vi "Error Process.vi"(8 "error in (no error)":errorcluster, 11 "View Model":T1) -> (0 "error out":errorcluster)   [LabVIEW 2013]
doc: "Responsible for collecting and handling all errors."
uses:
  View Model/Controls/View Model.ctl
  Controls/Error Model.ctl
  Controls/Error Types.ctl
  View Model/Controls/Shared Model.ctl
  Elevator Controller/Controls/Elevator Model.ctl
  Elevator Controller/Controls/Controller Overhead.ctl
  Elevator Controller/Controls/Elevator States.ctl
  Elevator Controller/Controls/Elevator Location.ctl
  Elevator Controller/Controls/Elevator Command Event.ctl
  Elevator Controller/Controls/Elevator Commands.ctl
  Configuration/Controls/Configuration Model.ctl
  Configuration/Controls/Configuration Data.ctl
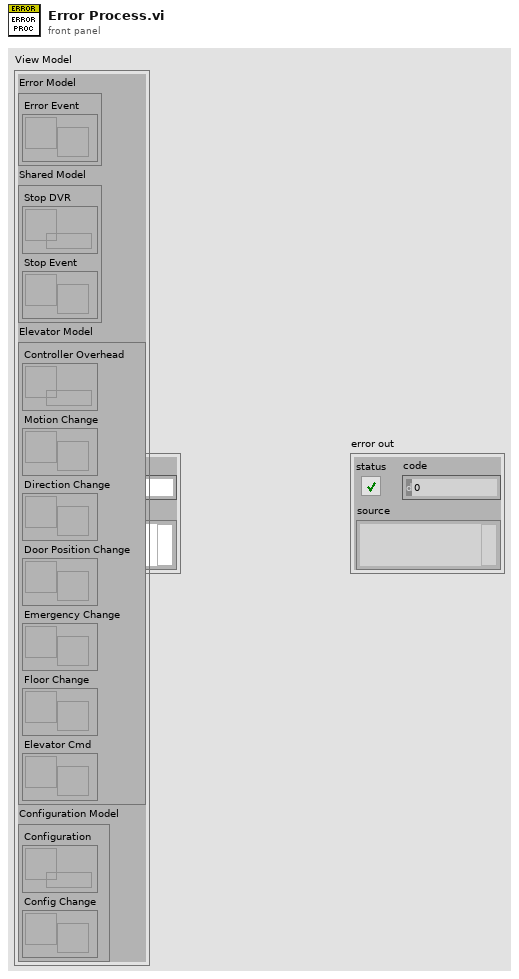
[diagram p1: front panel]
types:
  T1 = typedef "View Model.ctl" = cluster{"Error Model":T2, "Shared Model":T3, "Elevator Model":T4, "Configuration Model":T5}
  T2 = typedef "Error Model.ctl" = cluster{"Error Event":refnum<user-event>}
  T3 = typedef "Shared Model.ctl" = cluster{"Stop DVR":refnum<data-value>, "Stop Event":refnum<user-event>}
  T4 = typedef "Elevator Model.ctl" = cluster{"Controller Overhead":refnum<data-value>, "Motion Change":refnum<user-event>, "Direction Change":refnum<user-event>, "Door Position Change":refnum<user-event>, "Emergency Change":refnum<user-event>, "Floor Change":refnum<user-event>, "Elevator Cmd":refnum<user-event>}
  T5 = typedef "Configuration Model.ctl" = cluster{"Configuration":refnum<data-value>, "Config Change":refnum<user-event>}
  T6 = typedef "Error Types.ctl" = enum16{"Console Error", "Process Step Error", "Sensor Interface IO Error"}
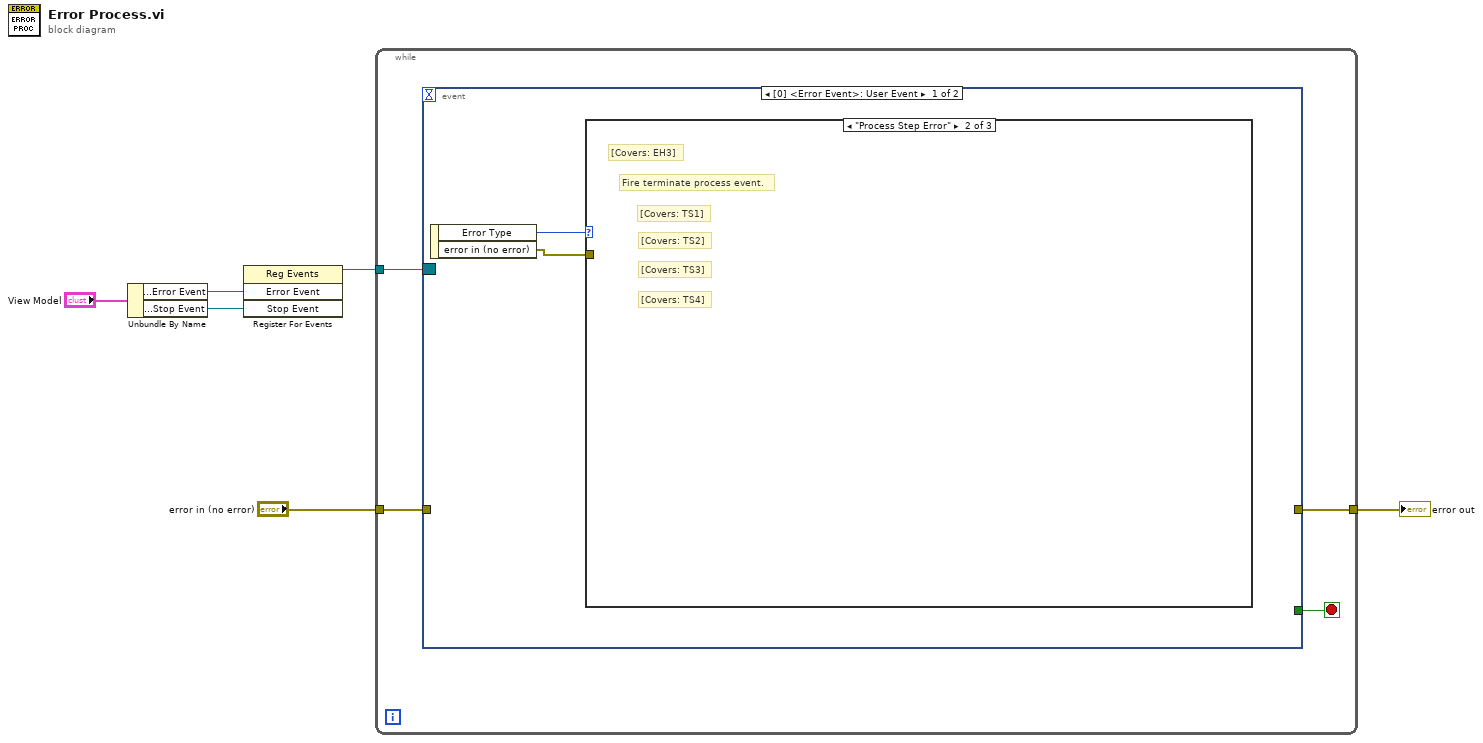
[diagram p0: block diagram]
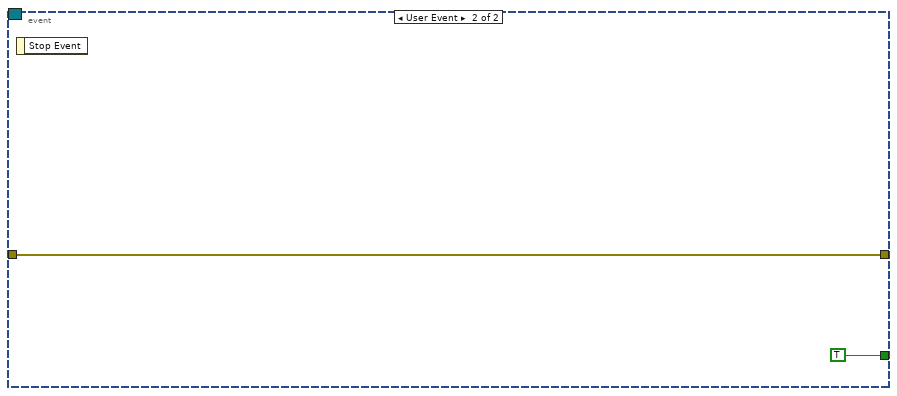
[diagram p4: hidden frame]
diagram:
  n1 = Unbundle By Name("View Model") -> ("Error Model.Error Event"=w5:refnum<user-event>, "Shared Model.Stop Event"=w3:refnum<user-event>)
  n2 = register-events(w5, w3) -> (reference out=w4:refnum<event-registration>)  [unwired: 2 in, 1 out]
  n3 = while {
    tunnel: w4 -> [w10]
    tunnel: "error in (no error)" -> [w8]
    tunnel: [w7] -> w1
    stop <- w9 stop-if-true
    n4 = event shown="[0] <Error Event>: User Event" {
      selector: w10 -> [_ _]
      dyn-events: _ -> [_ _]
      timeout: _ -> [_ _]
      tunnel: [_ TRUE] -> w9
      tunnel: w8 -> [_ w13]
      tunnel: [_ w13] -> w7
      event User Event {
        n5 = event-data() -> ("Error Type"=w12:T6, "error in (no error)"=w11:errorcluster)  [unwired: 1 in]
        n6 = case shown="\"Process Step Error\"" w12 {
          tunnel: w11 -> [_ _ _]
          frame "Console Error", Default {
            # "[Covers: EH1]"
            # "[Covers: EH1B]"
            # "[Covers: EH1A]"
            # "Console Error: Alert user.\nIf error source = Display Console View, notify user and clear\nerror.\n\nIf error source = User Console View, Allow user to choose to\nclear or continue w/ error. \n- If error cleared, continue last operation.\n- If continue, process error as a \"Process Step Error\""
          }
          frame "Process Step Error" {
            # "[Covers: TS4]"
            # "[Covers: TS3]"
            # "[Covers: TS2]"
            # "[Covers: TS1]"
            # "Fire terminate process event."
            # "[Covers: EH3]"
          }
          frame "Sensor Interface IO Error" {
            # "[Covers: EH4]"
          }
        }
      }
      event User Event {
        n7 = event-data() -> ()  [unwired: 1 in, 1 out]
      }
    }
  }
  "error out" <- w1
